vi "Emballage_BDD_GVF_PortCom.vi"(0 "Énum":enum16{"get", "set"}(ring), 1 "Imprimante certif. IN":string, 2 "PortCom Scanner IN":refnum<visa-resource-name>, 5 "PortCom imprimante IN":refnum<visa-resource-name>, 7 "Imprimante Zebra IN":string, 9 "bdd":bool, 11 "Error in":errorcluster caption="Error in (no error)", 12 "DecDroit_IN":string) -> (3 "Imprimante Zebra":string, 4 "PortCom Scanner":refnum<visa-resource-name>="COM3", 6 "PortCom imprimante OUT":refnum<visa-resource-name>="COM3", 10 "DecDroit_OUT":string, 13 "Imprimante Certif.":string, 14 "Result Set":string[][](array[string]), 15 "Error out":errorcluster)   [LabVIEW 2020]
uses:
  Modules/FS/60_FS_Controles/60_FS_SetGet.ctl
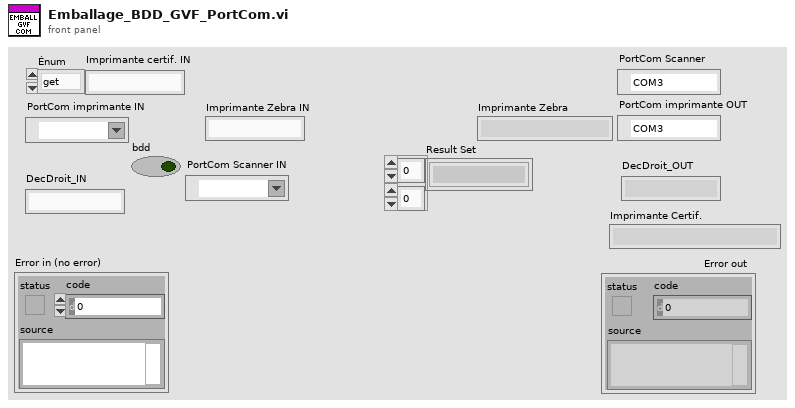
[diagram p1: front panel]
types:
  T1 = typedef "60_FS_SetGet.ctl" = enum16{"set", "get"}
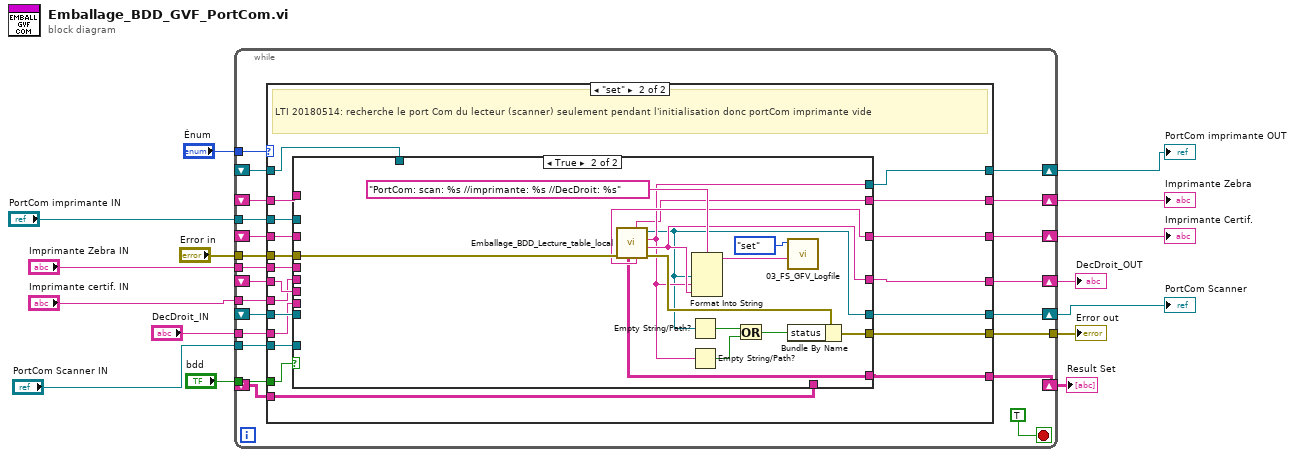
[diagram p0: block diagram]
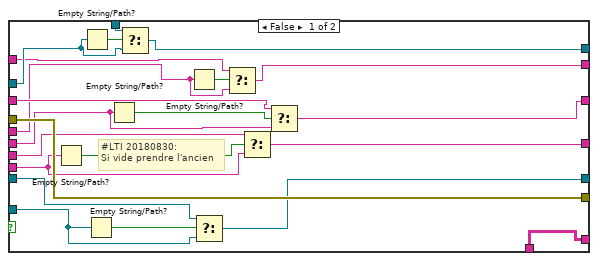
[diagram p3: hidden frame]
diagram:
  n1 = while {
    tunnel: "Énum" -> [w36]
    tunnel: "Error in" -> [w35]
    tunnel: [w34] -> w13
    shift-right: [w33] -> w12
    shift-left: _ -> [w32]
    shift-right: [w31] -> w11
    shift-left: _ -> [w30]
    tunnel: "bdd" -> [w29]
    tunnel: "PortCom imprimante IN" -> [w28]
    shift-right: [w27] -> w8
    shift-left: _ -> [w25]
    tunnel: "DecDroit_IN" -> [w26]
    shift-right: [w24] -> w6
    shift-left: _ -> [w23]
    tunnel: "Imprimante certif. IN" -> [w22]
    shift-right: [w21] -> w4
    shift-left: _ -> [w19]
    tunnel: "Imprimante Zebra IN" -> [w20]
    tunnel: "PortCom Scanner IN" -> [w18]
    shift-right: [w17] -> w1
    shift-left: _ -> [w16]
    stop <- TRUE stop-if-true
    n2 = case shown="\"set\"" w36 {
      tunnel: w35 -> [w44 w64]
      tunnel: [w44 w63] -> w34
      tunnel: [w41 w62] -> w33
      tunnel: w32 -> [w41 w58]
      tunnel: [w43 w61] -> w31
      tunnel: w30 -> [w43 w48]
      tunnel: w29 -> [_ w60]
      tunnel: w28 -> [_ w59]
      tunnel: [w42 w57] -> w27
      tunnel: w26 -> [_ w56]
      tunnel: w25 -> [w42 w55]
      tunnel: [w40 w54] -> w24
      tunnel: w23 -> [w40 w49]
      tunnel: w22 -> [_ w53]
      tunnel: [w39 w52] -> w21
      tunnel: w20 -> [_ w51]
      tunnel: w19 -> [w39 w47]
      tunnel: w18 -> [_ w50]
      tunnel: [w38 w46] -> w17
      tunnel: w16 -> [w38 w45]
      frame "get", Default {
      }
      frame "set" {
        # "LTI 20180514: recherche le port Com du lecteur (scanner) seulement pendant l'initialisation donc portCom imprimante vide"
        n3 = case shown="True" w60 {
          tunnel: w64 -> [w86 w94]
          tunnel: [w86 w101] -> w63
          tunnel: [w78 w89] -> w62
          tunnel: [w71 w90] -> w61
          tunnel: w59 -> [w73 _]
          tunnel: w58 -> [w80 _]
          tunnel: [w82 w91] -> w57
          tunnel: w56 -> [w83 _]
          tunnel: w55 -> [w84 _]
          tunnel: [w70 w92] -> w54
          tunnel: w53 -> [w76 _]
          tunnel: [w67 w88] -> w52
          tunnel: w51 -> [w68 _]
          tunnel: w50 -> [w79 _]
          tunnel: w49 -> [w75 _]
          tunnel: w48 -> [w72 _]
          tunnel: w47 -> [w66 _]
          tunnel: [w65 w87] -> w46
          tunnel: w45 -> [w65 _]
          frame False {
            # "#LTI 20180830:\nSi vide prendre l'ancien"
            n4 = Empty String/Path?(string/path=w83) -> (empty?=w85:bool)
            n5 = Empty String/Path?(string/path=w73) -> (empty?=w74:bool)
            n6 = Empty String/Path?(string/path=w79) -> (empty?=w81:bool)
            n7 = Empty String/Path?(string/path=w76) -> (empty?=w77:bool)
            n8 = Select(t=w72, s=w74, f=w73) -> (s? t:f=w71:refnum<visa-resource-name>)
            n9 = Empty String/Path?(string/path=w68) -> (empty?=w69:bool)
            n10 = Select(t=w80, s=w81, f=w79) -> (s? t:f=w78:refnum<visa-resource-name>)
            n11 = Select(t=w66, s=w69, f=w68) -> (s? t:f=w67:string)
            n12 = Select(t=w84, s=w85, f=w83) -> (s? t:f=w82:string)
            n13 = Select(t=w75, s=w77, f=w76) -> (s? t:f=w70:string)
          }
          frame True {
            n14 = call "Emballage_BDD_Lecture_table_local.vi"("entrée d'erreur (pas d'erreur)"=w94) -> ("sortie d'erreur"=w93:errorcluster, "Dec.Droite 2"=w91:string, "Com Imprimante"=w90:string, "Refnum VISA en sortie"=w89:refnum<visa-resource-name>, "Imprimante certif"=w92:string, "Imprimante Zebra"=w88:string, "Result Set"=w87:string[][])  [unwired: 4 in]
            n15 = Empty String/Path?(string/path=w89) -> (empty?=w99:bool)
            n16 = Empty String/Path?(string/path=w90) -> (empty?=w100:bool)
            n17 = Format Into String(format string="PortCom: scan: %s //imprimante: %s //DecDroit: %s", w89, w90, w91) -> (resulting string=w95:string)  [unwired: 2 in, 1 out]
            n18 = Or(x=w99, y=w100) -> (x .or. y?=w98:bool)
            n19 = call "03_FS_GFV_Logfile.vi"("Chaîne"=w95, "States"=60_FS_SetGet."set") -> ()  [unwired: 8 in, 2 out]
            n20 = Bundle By Name(cluster=w93, "status"=w98) -> (w101:errorcluster)
          }
        }
      }
    }
  }
  "Error out" <- w13
  "PortCom Scanner" <- w12
  "PortCom imprimante OUT" <- w11
  "DecDroit_OUT" <- w8
  "Imprimante Certif." <- w6
  "Imprimante Zebra" <- w4
  "Result Set" <- w1
